vi "Get All Parameters.vi"(8 "error in (no error)":errorcluster, 11 "Macro Step in":refnum<class "Macro Step.lvclass">) -> (0 "error out":errorcluster, 2 "Parameters":T1={"Type"=enum."Mouse Move", "X"=0, "Y"=0, "Delay"=0, "Key"=65, "Repeat"=0, "RClick?"=FALSE, "App/Window Name"="", "Notes"="", "Assertion Type"=enum."Control Position", "Control Name"="", "Disabled"=enum."Enabled", "Visible"=enum."Visible", "Left"=0, "Top"=0, "Width"=0, "Height"=0, "Expected Image"={"image type"=0, "image depth"=0, "image"=[], "mask"=[], "colors"=[], "Rectangle"={"left"=0, "top"=0, "right"=0, "bottom"=0}}}, 3 "Macro Step out":refnum<class "Macro Step.lvclass">)   [LabVIEW 2020, in "MacroAssert.lvlib" / "Macro Step.lvclass"]
uses:
  Macro Step.lvclass
  Macro Step.lvclass/Macro Step.ctl
  Step/Step.lvclass
  CTLs/Step V3.ctl
  MacroAssert.lvlib
  CTLs/Step Type V3.ctl
  CTLs/Assertion Type.ctl
  <vilib>/picture/picture.llb/imagedata.ctl
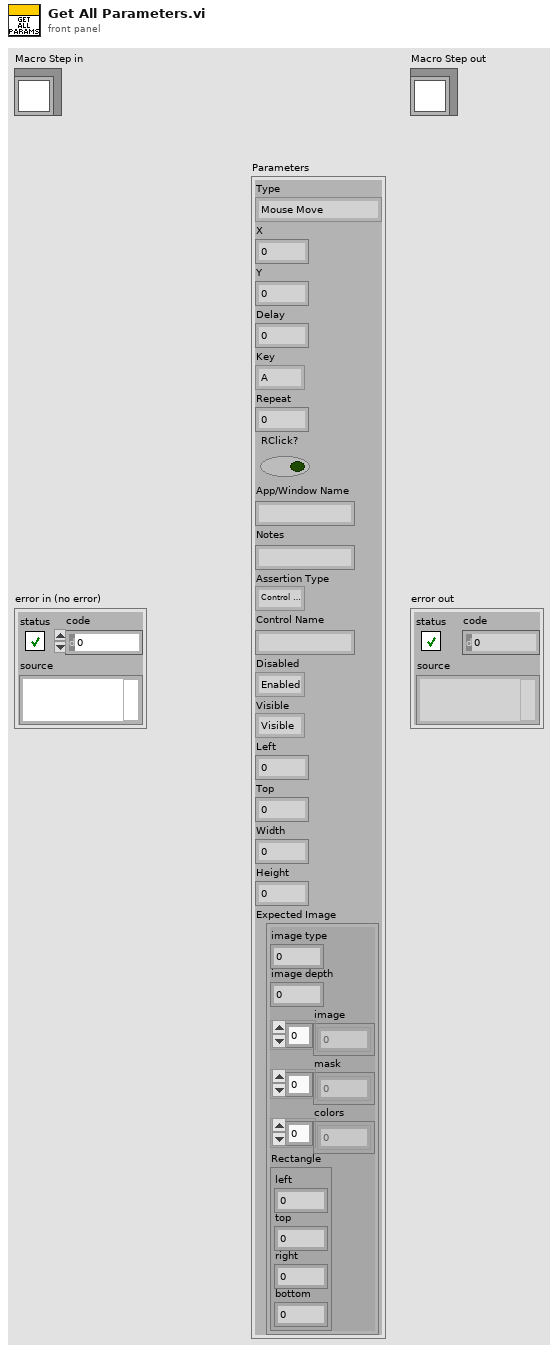
[diagram p1: front panel]
types:
  T1 = typedef "MacroAssert.lvlib/Step V3.ctl" = cluster{"Type":T2, "X":i32, "Y":i32, "Delay":i32, "Key":u8, "Repeat":i32, "RClick?":bool, "App/Window Name":string, "Notes":string, "Assertion Type":T3, "Control Name":string, "Disabled":enum8{"Enabled", "Disabled", "Disabled and Grayed Out"}, "Visible":enum16{"Visible", "Not Visible"}, "Left":i16, "Top":i16, "Width":i16, "Height":i16, "Expected Image":T4}
  T2 = typedef "MacroAssert.lvlib/Step Type V3.ctl" = enum16{"Mouse Move", "Mouse Click", "Key Press", "Wait", "Mouse Down", "Mouse Up", "Key Down", "Key Up", "Test Assertion", "Maximize Window", "Restore Window", "Minimize Window", "Close Window", "Bring Window to Front", "Send Window to Back"}
  T3 = typedef "MacroAssert.lvlib/Assertion Type.ctl" = enum16{"Control Position", "Control Visible", "Control Disabled", "Control Image"}
  T4 = typedef "imagedata.ctl" = cluster{"image type":i32, "image depth":i32, "image":u8[], "mask":u8[], "colors":u32[], "Rectangle":cluster{"left":i16, "top":i16, "right":i16, "bottom":i16}}
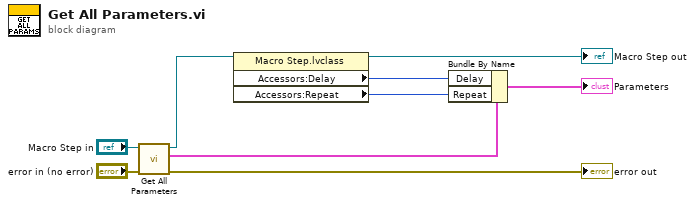
[diagram p0: block diagram]
diagram:
  n1 = call-parent "Get All Parameters.vi"("error in (no error)"="error in (no error)", "Step in"="Macro Step in") -> ("error out"=→"error out":errorcluster, "Parameters"=w8:T1, "Step out"=w7:refnum<class "Macro Step.lvclass">)  [unwired: 7 in]
  n2 = property class="Macro Step.lvclass"(reference=w7) -> (reference out=→"Macro Step out":refnum<class "Macro Step.lvclass">, "Accessors:Delay"=w2:i32, "Accessors:Repeat"=w1:i32)  [unwired: 1 in, 1 out]
  n3 = Bundle By Name(cluster=w8, "Delay"=w2, "Repeat"=w1) -> (→"Parameters":T1)
